vi "subrszvl_core_attribute_express.vi"(0 "instrument handle":refnum<visa-resource-name> caption="VISA resource name", 1 "Attribute ID":string, 2 "Attribute Operation":u16(ring)=1 items=["Read", "Write", "Read Direct", "Write Direct", "Write Fix", "Compose Direct", "Compose Fix"], 3 "SCPI Command":string, 4 "Direct cmd in":string, 5 "error in (no error)":errorcluster, 6 "Input I32":i32, 8 "Input Double":dbl format="%#_6p", 10 "Input String":string, 12 "Input Boolean":bool, 15 "Repeated Capabilities":string, 17 "Input I64":i64) -> (7 "Output I32":i32, 9 "Output Double":dbl, 11 "Output String":string, 13 "Output Boolean":bool, 14 "instrument handle out":refnum<visa-resource-name> caption="VISA resource name", 16 "Output I64":i64, 18 "Direct cmd out":string, 19 "error out":errorcluster)   [LabVIEW 2014]
uses:
  rszvl_rsidr_core.lvlib
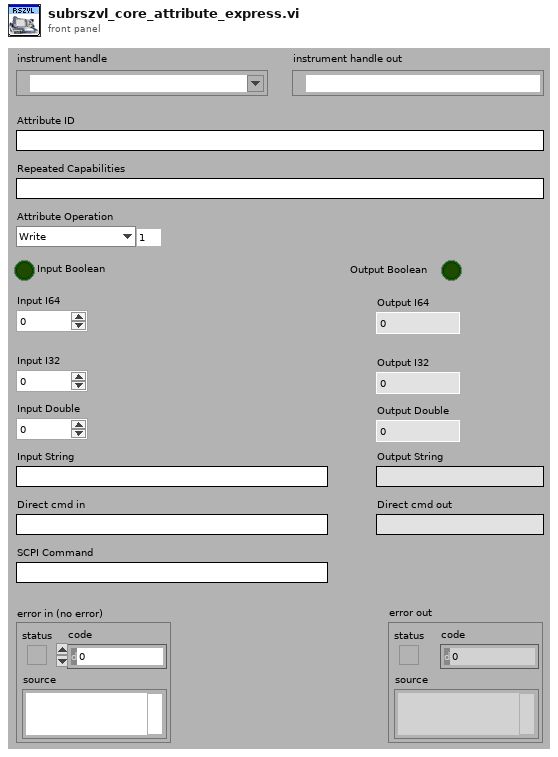
[diagram p1: front panel]
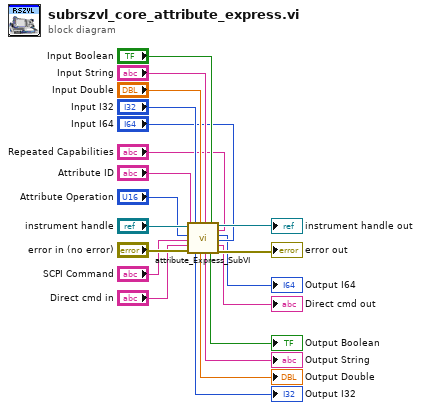
[diagram p0: block diagram]
diagram:
  n1 = call "attribute_Express_SubVI.vi"("VISA resource name"="instrument handle", "Attribute ID"="Attribute ID", "Attribute Operation"="Attribute Operation", "SCPI Command"="SCPI Command", "Direct cmd in"="Direct cmd in", "error in (no error)"="error in (no error)", "Input I32"="Input I32", "Input Double"="Input Double", "Input String"="Input String", "Input Boolean"="Input Boolean", "Repeated Capabilities"="Repeated Capabilities", "Input I64"="Input I64") -> ("Output I32"=→"Output I32":i32, "Output Double"=→"Output Double":dbl, "Output String"=→"Output String":string, "Output Boolean"=→"Output Boolean":bool, "VISA resource name out"=→"instrument handle out":refnum<visa-resource-name>, "Output I64"=→"Output I64":i64, "Direct cmd out"=→"Direct cmd out":string, "error out"=→"error out":errorcluster)
